vi "FTP_ReplyCheck.vi"(0 "expected class":T1(ring)=enum."500 - Permanent", 1 "reply":i32) -> (3 "match":bool, 4 "class":T1(ring)=enum."500 - Permanent", 5 "sub class":u16(ring) items=["Syntax", "Information", "Connection", "Authentication", "Unspecified", "File System", "unknown"], 6 "code":i32)   [LabVIEW 2012]
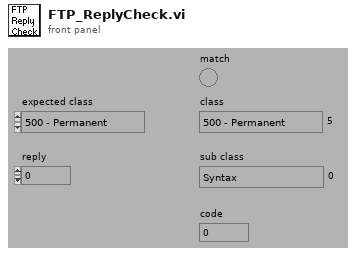
[diagram p1: front panel]
types:
  T1 = enum16{"unknown", "100 + Prelim", "200 + ", "300 + Intermed", "400 - Transient", "500 - Permanent"}
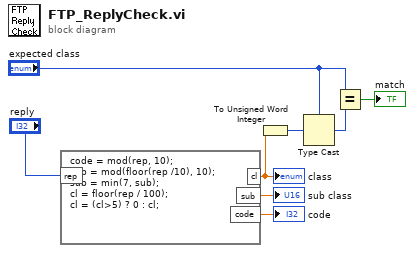
[diagram p0: block diagram]
diagram:
  n1 = formula code="code = mod(rep, 10);\nsub = mod(floor(rep /10), 10);\nsub = min(7, sub);\ncl = floor(rep / 100);\ncl = (cl>5) ? 0 : cl;"("rep"="reply") -> ("cl"=w5:dbl, "sub"=→"sub class":dbl, "code"=→"code":dbl)
  "class" <- w5
  n2 = To Unsigned Word Integer(number=w5) -> (unsigned 16bit integer=w1:u16)
  n3 = Type Cast(type="expected class", x=w1) -> (*(type *) &x=w3:T1)
  n4 = Equal?(x="expected class", y=w3) -> (x = y?=→"match":bool)
